vi "number from rotated float string (SubVI).vi"(5 "String":string) -> (0 "float number":sgl, 1 "Rotated Float String":string, 2 "rotated float number":sgl)   [LabVIEW 2017, in "LV_Unicorn.lvlib"]
uses:
  LV_Unicorn.lvlib
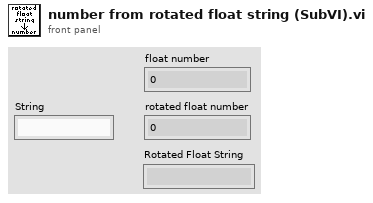
[diagram p1: front panel]
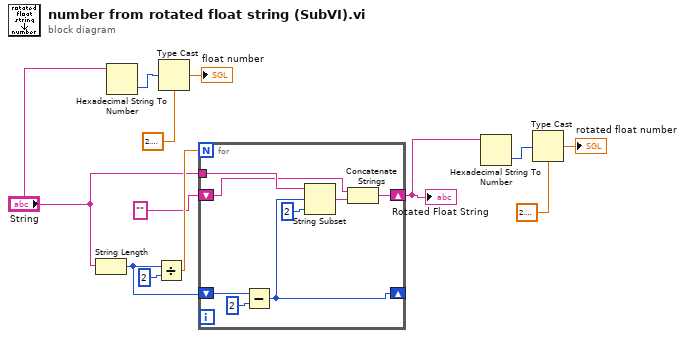
[diagram p0: block diagram]
diagram:
  n1 = String Length(string="String") -> (length=w9:i32)
  n2 = Hexadecimal String To Number(string="String") -> (number=w2:u32)  [unwired: 2 in, 1 out]
  n3 = Divide(x=w9, y=2) -> (x/y=w11:dbl)
  n4 = Type Cast(type=sgl 2.3, x=w2) -> (*(type *) &x=→"float number":sgl)
  n5 = for {
    N: w11 -> [_]
    tunnel: "String" -> [w20]
    shift-right: [w13] -> _
    shift-left: w9 -> [w19]
    shift-right: [w14] -> w7
    shift-left: "" -> [w16]
    n6 = Subtract(x=w19, y=2) -> (x-y=w13:i32)
    n7 = String Subset(string=w20, offset (0)=w13, length (rest)=2 ("length (rest)")) -> (substring=w15:string)
    n8 = Concatenate Strings(w16, w15) -> (w14:string)
  }
  "Rotated Float String" <- w7
  n9 = Hexadecimal String To Number(string=w7) -> (number=w5:u32)  [unwired: 2 in, 1 out]
  n10 = Type Cast(type=sgl 2.3, x=w5) -> (*(type *) &x=→"rotated float number":sgl)
